vi "DuplicateItem.vi"(8 "error in (no error)":errorcluster, 11 "PLC_Module in":refnum<class "PLC_Module.lvclass">) -> (0 "error out":errorcluster, 3 "PLC_Module out":refnum<class "PLC_Module.lvclass">)   [LabVIEW 2025, in "PLC_Module.lvlib" / "PLC_Module.lvclass"]
uses:
  PLC_Module.lvclass
  PLC_Module.lvclass/PLC_Module.ctl
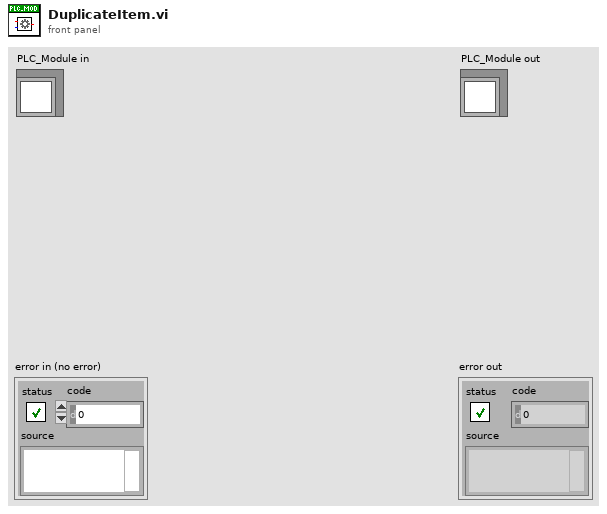
[diagram p1: front panel]
types:
  T1 = typedef "PLC_Module.lvlib/PLC_Module.lvclass/PLC_Data_Config.ctl" = map{string, cluster{"Config":T2, "Get Value":string, "Set Value":string}}
  T2 = typedef "PLC_Module.lvlib/PLC_Module.lvclass/PLC_Data.ctl" = cluster{"Address":string, "Direction":enum16{"PC->PLC", "PLC->PC"}, "DataType":T3, "Description":string}
  T3 = typedef "PLC_Module.lvlib/PLC_Module.lvclass/PLC_Data_Type.ctl" = enum16{"Boolean", "Single Float", "U8", "U32", "U32_Array", "String"}
  T4 = cluster{"Config":T2, "Get Value":string, "Set Value":string}
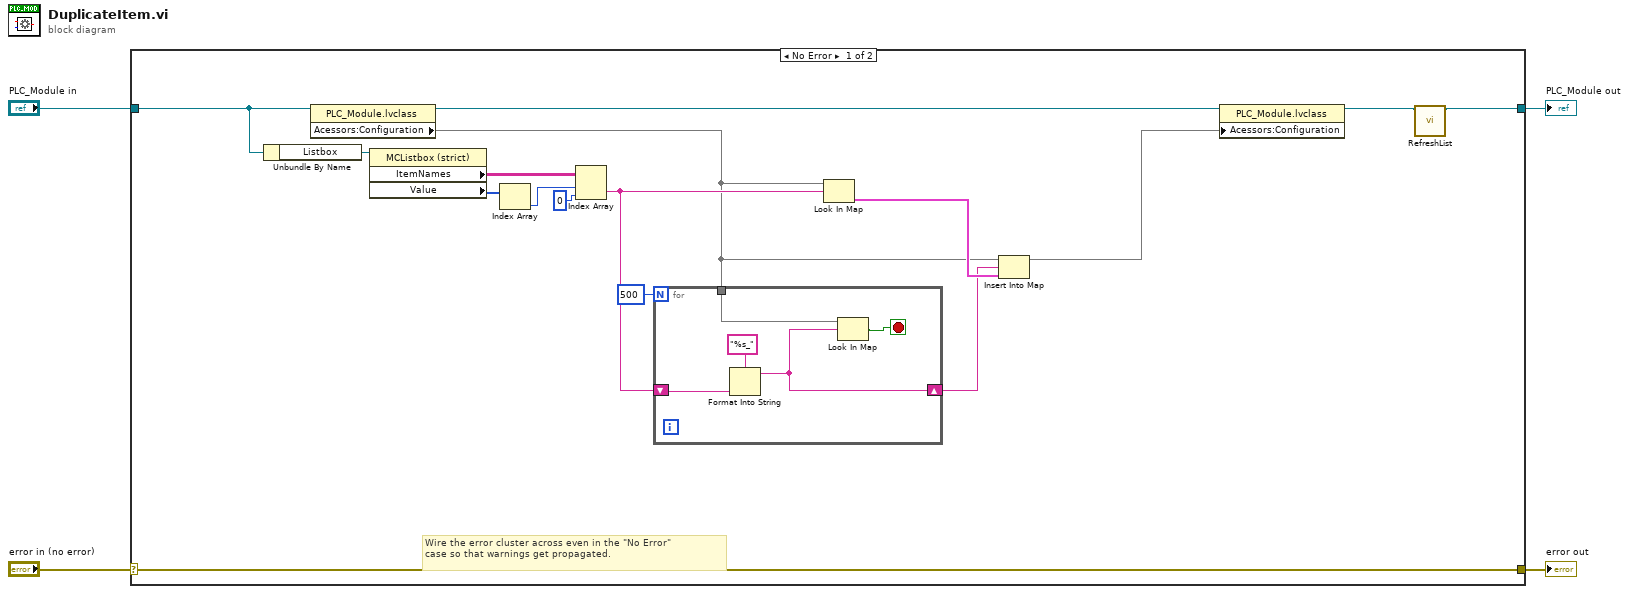
[diagram p0: block diagram]
diagram:
  n1 = case shown="No Error" "error in (no error)" {
    selector: "error in (no error)" -> [w20 w27]
    tunnel: [w20 w27] -> w3
    tunnel: [w9 w26] -> w1
    tunnel: "PLC_Module in" -> [w19 w26]
    frame No Error {
      # "Wire the error cluster across even in the \"No Error\"\ncase so that warnings get propagated."
      n2 = Unbundle By Name(w19) -> ("Listbox"=w18:refnum<vi>)
      n3 = property class="PLC_Module.lvclass"(reference=w19) -> (reference out=w13:refnum<class "PLC_Module.lvclass">, "Acessors:Configuration"=w7:T1)  [unwired: 1 in, 1 out]
      n4 = property class="MCListbox (strict)"(reference=w18) -> ("ItemNames"=w17:string[][], "Value"=w15:i32[])  [unwired: 1 in, 2 out]
      n5 = Index Array(array=w15) -> (element=w14:i32)  [unwired: 1 in]
      n6 = Index Array(array=w17, index (row)=w14, index (col)=0 ("disabled index (col)")) -> (element=w8:string)
      n7 = for {
        N: 500 -> [_]
        tunnel: w7 -> [w23]
        shift-right: [w21] -> w6
        shift-left: w8 -> [w25]
        stop <- w22 stop-if-true
        n8 = Format Into String(format string="%s_", w25) -> (resulting string=w21:string)  [unwired: 2 in, 1 out]
        n9 = Look In Map(map=w23, key=w21) -> (key not found?=w22:bool)  [unwired: 1 in, 1 out]
      }
      n10 = Look In Map(map=w7, key=w8) -> (value=w12:T4)  [unwired: 1 in, 1 out]
      n11 = Insert Into Map(map in=w7, key=w6, value=w12) -> (map out=w11:T1)  [unwired: 2 out]
      n12 = property class="PLC_Module.lvclass"(reference=w13, "Acessors:Configuration"=w11) -> (reference out=w10:refnum<class "PLC_Module.lvclass">)  [unwired: 1 in, 1 out]
      n13 = call "RefreshList.vi"("PLC_Module in"=w10) -> ("PLC_Module out"=w9:refnum<class "PLC_Module.lvclass">)  [unwired: 9 in, 1 out]
    }
    frame Error {
    }
  }
  "error out" <- w3
  "PLC_Module out" <- w1
